vi "DBM Initialize.vi"(8 "에러 입력":errorcluster caption="에러 입력(에러 없음)") -> (0 "에러 출력":errorcluster, 2 "STD List":string[](array[string]), 3 "Func List":string[][](array[string]), 4 "항목명":string[](array[string]), 5 "교정기능목록":string[][](array[string]), 6 "모델요청 List":string[][](array[string]), 7 "세부분류목록":string[][](array[string]))   [LabVIEW 2020]
uses:
  Controls/Cmd_Read Query.ctl
  Public/Polymorph/Array Dedup_2D Str.vi
  <vilib>/addons/database/NI_Database_API.lvlib
panel:
  out "속성목록":cluster{"문자열":string, "문자열":string}[](array[cluster])
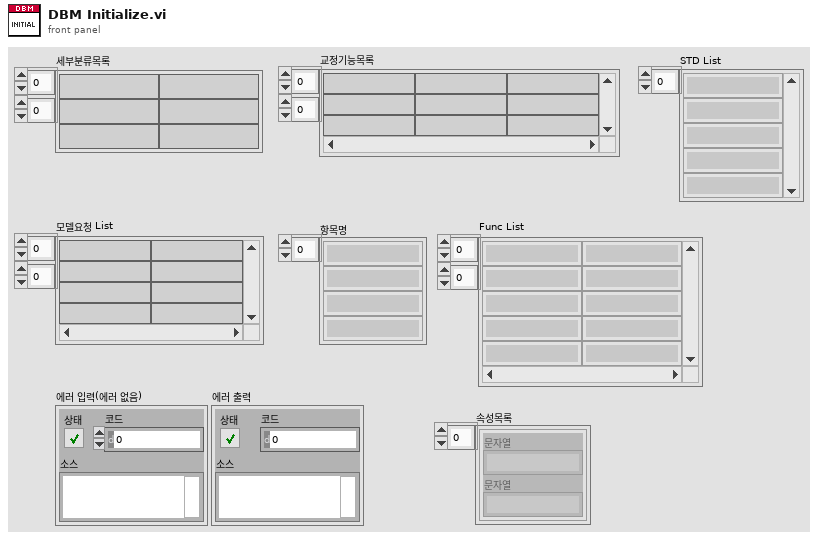
[diagram p1: front panel]
types:
  T1 = typedef "Cmd_Read Query.ctl" = enum16{"교정자 이름 얻기", "인증교정자 얻기", "기술책임자 얻기", "기책부책 얻기", "등록번호 얻기", "등록정보 얻기", "업체정보 얻기", "교정일자(CAMAS) 얻기", "교정일자(CALSTD) 얻기", "교정환경 얻기", "교정절차서 목록 얻기", "교정절차서명 얻기", "교정절차 목록얻기", "교정절차 얻기", "PROC 교정절차 얻기", "PROC SPEC 얻기", "교정절차(Func별) 얻기", "교정절차(Func_ext별) 얻기", "기관코드 얻기", "교정기능(세부분류) 얻기", "교정기능(모델) 얻기", "교정기능 목록 얻기", "교정기능 명칭 얻기", "교정기능 항목명칭 얻기", "DB (사용기준기) 얻기", "DB (기준기이름) 얻기", "DB (기준기이름목록) 얻기", "DB (기준기목록) 얻기", "DB (기준기값) 얻기", "DB (CMC) 얻기", "DB (FUNC) 얻기", "DB (CALNAME) 얻기", "DB (STDNAME) 얻기", "DB (SPEC) 얻기", "모델(항목전체) 얻기", "모델(최대범위) 얻기", "모델(최소범위) 얻기", "모델(최대최소) 얻기", "모델(범위조건) 얻기", "모델(등록요청) 얻기", "모델(형식별) 얻기", "모델(조건별) 얻기", "모델(모델검색) 얻기", "세부분류 목록 얻기", "기준기등록리스트 얻기", "STD Cal Date Check", "DB등록일자 얻기", "적용항목 얻기", "기타정보 얻기", "기준기요청 얻기", "서버버전 얻기"}
  T2 = typedef "NI_Database_API.lvlib/Conn ObjectReference.ctl" = refnum<k1>
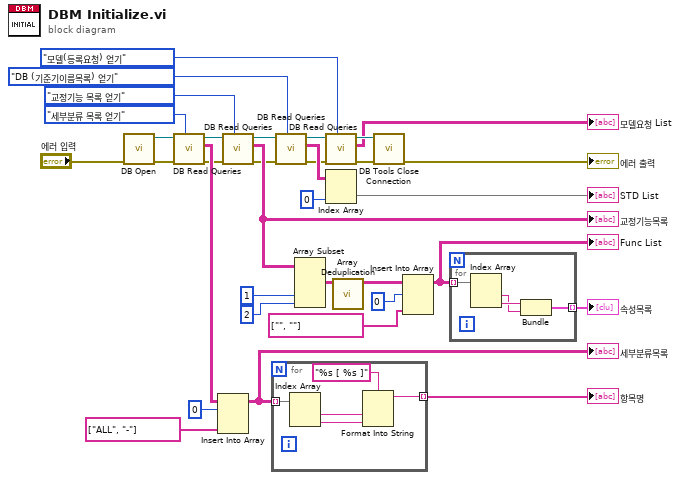
[diagram p0: block diagram]
diagram:
  n1 = call "DB Open.vi"("에러 입력"="에러 입력") -> ("에러 출력"=w26:errorcluster, "참조 번호 출력"=w27:T2)  [unwired: 9 in]
  n2 = call "DB Read Queries.vi"("Query Command"=Cmd_Read_Query."세부분류 목록 얻기", "에러 입력(에러 없음)"=w26, "참조 번호 입력"=w27) -> ("에러 출력"=w25:errorcluster, "Data"=w31:string[][], "참조 번호 출력"=w24:T2)  [unwired: 4 in, 2 out]
  n3 = Insert Into Array(array=w31, index (row)=0 ("인덱스 (행)"), new element=string[] ["ALL", "-"] ("새 원소/부분배열")) -> (w2:string[][])  [unwired: 1 in]
  "세부분류목록" <- w2
  n4 = call "DB Read Queries.vi"("Query Command"=Cmd_Read_Query."교정기능 목록 얻기", "에러 입력(에러 없음)"=w25, "참조 번호 입력"=w24) -> ("에러 출력"=w1:errorcluster, "Data"=w22:string[][], "참조 번호 출력"=w12:T2)  [unwired: 4 in, 2 out]
  "교정기능목록" <- w22
  n5 = for {
    tunnel: w2 -> [w39] mode=indexing
    tunnel: [w35] -> w30 mode=indexing
    n6 = Index Array(array=w39) -> (element #1=w36:string, element #2=w38:string)  [unwired: 2 in]
    n7 = Format Into String(format string="%s [ %s ]" ("포맷 문자열"), w36, w38) -> (resulting string=w35:string)  [unwired: 2 in, 1 out]
  }
  "항목명" <- w30
  n8 = call "DB Read Queries.vi"("Query Command"=Cmd_Read_Query."DB (기준기이름목록) 얻기", "에러 입력(에러 없음)"=w1, "참조 번호 입력"=w12) -> ("에러 출력"=w9:errorcluster, "Data"=w14:string[][], "참조 번호 출력"=w8:T2)  [unwired: 4 in, 2 out]
  n9 = Array Subset(array=w22, index (col)=1 ("비활성화된 인덱스 (열)"), length (col)=2 ("길이")) -> (w21:string[][])  [unwired: 2 in]
  n10 = call "DB Read Queries.vi"("Query Command"=Cmd_Read_Query."모델(등록요청) 얻기", "에러 입력(에러 없음)"=w9, "참조 번호 입력"=w8) -> ("에러 출력"=w6:errorcluster, "Data"=→"모델요청 List":string[][], "참조 번호 출력"=w7:T2)  [unwired: 4 in, 2 out]
  n11 = Index Array(array=w14, index (col)=0 ("비활성화된 인덱스 (열)")) -> (element=→"STD List":string[])  [unwired: 1 in]
  n12 = call-poly "Array Deduplication.vi"("배열 in"=w21) -> ("배열 out"=w17:string[][])  [unwired: 9 in, 1 out]
  n13 = call <vilib>:"DB Tools Close Connection.vi"("error in (no error)"=w6, "connection reference"=w7) -> ("error out"=→"에러 출력":errorcluster)  [unwired: 5 in]
  n14 = Insert Into Array(array=w17, index (row)=0 ("인덱스 (행)"), new element=string[] ["", ""] ("새 원소/부분배열")) -> (w3:string[][])  [unwired: 1 in]
  "Func List" <- w3
  n15 = for {
    tunnel: w3 -> [w43] mode=indexing
    tunnel: [w42] -> w18 mode=indexing
    n16 = Index Array(array=w43) -> (element #1=w40:string, element #2=w41:string)  [unwired: 2 in]
    n17 = Bundle("문자열"=w41, "문자열"=w40) -> (w42:cluster{"문자열":string, "문자열":string})  [unwired: 1 in]
  }
  "속성목록" <- w18
